vi "PH_ImageCoG_Plotter.export Data.vi"(0 "i ref in":refnum<vi>, 5 "error in (no error)":errorcluster) -> (14 "i ref out":refnum<vi>, 19 "error out":errorcluster)   [LabVIEW 2014, in "PH_ImageCoG_Plotter.lvlib"]
doc: "This VI exports data to a file"
uses:
  PH_ImageCoG_Plotter.lvlib
  PH_Basics/PH_Img_BaseClass/PH_Img_BaseClass.lvlib
  PH_Basics/PH_Common/PH_Common.lvlib
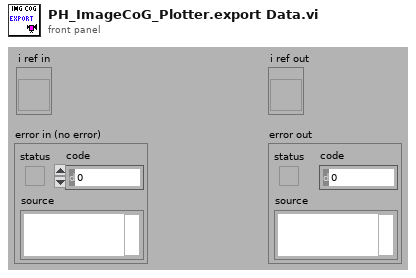
[diagram p1: front panel]
types:
  T1 = typedef "PH_ImageCoG_Plotter.lvlib/PH_ImageCoG_Plotter.i attribute.ctl" = cluster{"GUI Refs":cluster{"Delete":refnum<vi>, "Calibration status":refnum<vi>, "BI subtracted":refnum<vi>, "calc Beam Anal":refnum<vi>, "CoG - x":refnum<vi>, "CoG - y":refnum<vi>, "Type":refnum<vi>, "Center":refnum<vi>, "exp - X":refnum<vi>, "exp - Y":refnum<vi>, "Delta - X":refnum<vi>, "Delta - Y":refnum<vi>, "Available Cams":refnum<vi>, "CoG X":refnum<vi>, "CoG Y":refnum<vi>, "Delta X":refnum<vi>, "Delta Y":refnum<vi>, "Export Data":refnum<vi>, "Calibration data":refnum<vi>}, "Calibration":cluster{"Status":T2, "Calibration data":T3, "Calibration Data File":path}, "Beam Analysis":cluster{"on":bool, "exp - X":i32, "exp - Y":i32, "Type":bool, "Data":cluster{"current time":timestamp, "CoG-x":dbl, "CoG-y":dbl, "Delta-x":dbl, "Delta-y":dbl}[], "Datasets strored":i32, "Dataarray Size":i32}, "Cam instances":string[], "DIM Service Events":T4[], "Images":cluster{"Background":T7, "OP":T7, "GUI":T7}}
  T2 = typedef "PH_StatusHandler.lvlib/PH_StatusHandler.Status.ctl" = i16
  T3 = typedef "PH_ImageCalibrator.lvlib/PH_ImageCalibrator.Calibration Data.ctl" = cluster{"Date":string, "Time":string, "Cam Settings":cluster{"Cam ID":string, "Gain":dbl, "Brightness":dbl, "Shutter":dbl, "Cam Error":bool, "Mode":i32}, "Background Image":cluster{"Image":dbl[][], "Image Error":bool}, "Linear Calibration":cluster{"Calibration Factor":dbl, "not mm or mrad":bool}, "Energy Calibration":cluster{"Calibration Factor":dbl, "no mJ":bool}}
  T4 = typedef "BaseProcess.lvlib/BaseProcess.event definition.ctl" = cluster{"CAEEvtDef":T5, "Data Descriptor":T6}
  T5 = typedef "CAEObj.lvlib/CAEObj.event definition.ctl" = cluster{"URL":string, "enable":bool, "ignoreResID":bool}
  T6 = typedef "BaseProcess.lvlib/BaseProcess.descriptor string definition.ctl" = string
  T7 = typedef "IMAQ Image.ctl" = refnum<image>
  T8 = cluster{"current time":timestamp, "CoG-x":dbl, "CoG-y":dbl, "Delta-x":dbl, "Delta-y":dbl}[]
  T9 = cluster{"current time":timestamp, "CoG-x":dbl, "CoG-y":dbl, "Delta-x":dbl, "Delta-y":dbl}
  T10 = typedef "PH_Img_BaseClass.lvlib/PH_Img_BaseClass.i attribute.ctl" = cluster{"GUI Refs":T11, "Timeout Image [ms]":i32, "Default Periodic Period [ms]":i32, "Camera":cluster{"Instancename":string, "Notifier":refnum<notifier>}, "Palette":T12, "Cam Settings":cluster{"Cam ID":string, "Gain":dbl, "Brightness":dbl, "Shutter":dbl, "Cam Info Failure":bool, "Mode":i32}}
  T11 = typedef "PH_Img_BaseClass.lvlib/PH_Img_BaseClass.GUI Refs.ctl" = cluster{"Timeout":refnum<vi>, "Image":refnum<vi>, "Palette":refnum<vi>, "Timeout Set":refnum<vi>}
  T12 = typedef "PH_Img_BaseClass.lvlib/PH_Img_BaseClass.Palette.ctl" = i32
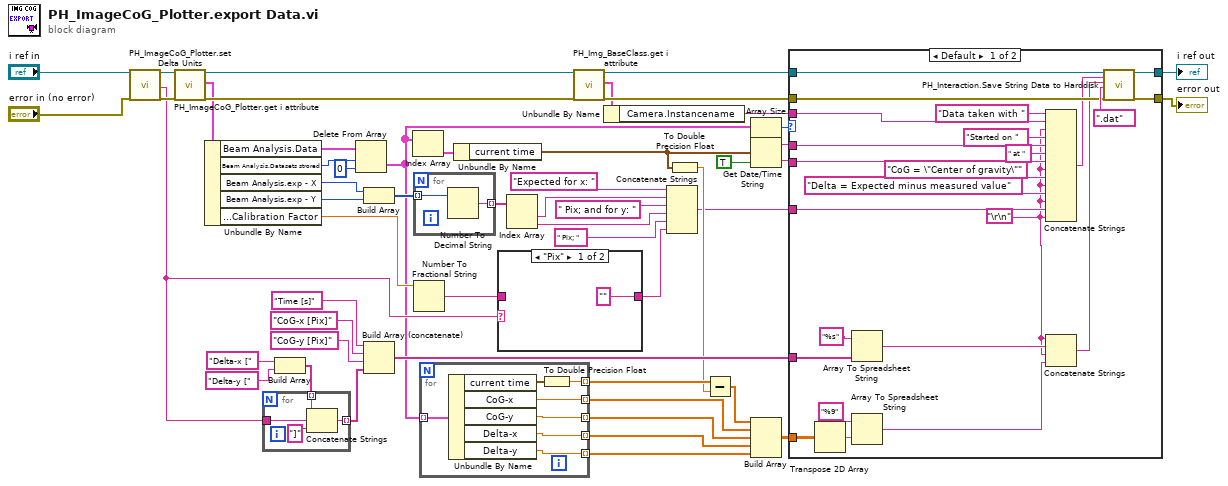
[diagram p0: block diagram]
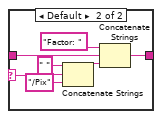
[diagram p2: hidden frame]
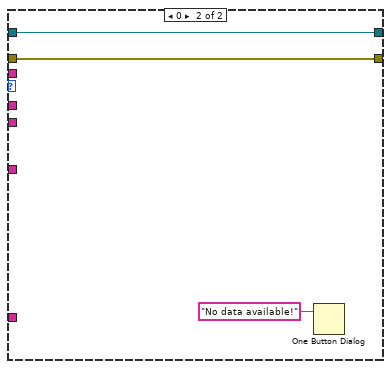
[diagram p3: hidden frame]
diagram:
  n1 = call "PH_ImageCoG_Plotter.set Delta Units.vi"("i ref in"="i ref in", "error in (no error)"="error in (no error)") -> ("i ref out"=w44:refnum<vi>, "Unit"=w10:string, "error out"=w42:errorcluster)  [unwired: 15 in]
  n2 = call "PH_ImageCoG_Plotter.get i attribute.vi"("i ref in"=w44, "error in (no error)"=w42) -> ("i ref out"=w5:refnum<vi>, "i attribute"=w51:T1, "error out"=w52:errorcluster)  [unwired: 15 in]
  n3 = Unbundle By Name(w51) -> ("Beam Analysis.Data"=w33:T8, "Beam Analysis.Datasets strored"=w8:i32, "Beam Analysis.exp - X"=w22:i32, "Beam Analysis.exp - Y"=w23:i32, "Calibration.Calibration data.Linear Calibration.Calibration Factor"=w20:dbl)
  n4 = Build Array("Delta-x [" ("element"), "Delta-y [" ("element")) -> (w35:string[])
  n5 = for {
    tunnel: w10 -> [w57]
    tunnel: w35 -> [w55] mode=indexing
    tunnel: [w54] -> w34 mode=indexing
    n6 = Concatenate Strings(w55, w57, "]" ("string")) -> (w54:string)
  }
  n7 = Delete From Array(array=w33, length=w8, index=0) -> (deleted portion=w9:T8)  [unwired: 1 out]
  n8 = Build Array(w22, w23) -> (w21:i32[])
  n9 = Build Array (concatenate)("Time [s]" ("format string"), "CoG-x [Pix]" ("element"), "CoG-y [Pix]" ("element"), w34) -> (w41:string[])
  n10 = Index Array(array=w9) -> (element=w50:T9)  [unwired: 1 in]
  n11 = for {
    tunnel: w21 -> [w59] mode=indexing
    tunnel: [w58] -> w18 mode=indexing
    n12 = Number To Decimal String(number=w59) -> (decimal integer string=w58:string)  [unwired: 1 in]
  }
  n13 = Number To Fractional String(number=w20) -> (F-format string=w12:string)  [unwired: 3 in]
  n14 = for {
    tunnel: w9 -> [w66] mode=indexing
    tunnel: [w64] -> w32 mode=indexing
    tunnel: [w63] -> w28 mode=indexing
    tunnel: [w62] -> w27 mode=indexing
    tunnel: [w61] -> w26 mode=indexing
    tunnel: [w60] -> w25 mode=indexing
    n15 = Unbundle By Name(w66) -> ("current time"=w65:timestamp, "CoG-x"=w63:dbl, "CoG-y"=w62:dbl, "Delta-x"=w61:dbl, "Delta-y"=w60:dbl)
    n16 = To Double Precision Float(number=w65) -> (double precision float=w64:dbl)
  }
  n17 = Unbundle By Name(w50) -> ("current time"=w31:timestamp)
  n18 = case shown="\"Pix\"" w10 {
    selector: w10 -> [_ w69]
    tunnel: ["" w74] -> w13
    tunnel: w12 -> [_ w72]
    frame "Pix" {
    }
    frame Default {
      n19 = Concatenate Strings(" " ("string"), w69, "/Pix" ("string")) -> (w71:string)
      n20 = Concatenate Strings("Factor: " ("string"), w72, w71) -> (w74:string)
    }
  }
  n21 = Index Array(array=w18) -> (element #1=w17:string, element #2=w15:string)  [unwired: 2 in]
  n22 = call "PH_Img_BaseClass.get i attribute.vi"("i ref in"=w5, "error in (no error)"=w52) -> ("i ref out"=w2:refnum<vi>, "i attribute"=w4:T10, "error out"=w6:errorcluster)  [unwired: 15 in]
  n23 = Unbundle By Name(w4) -> ("Camera.Instancename"=w3:string)
  n24 = Concatenate Strings("Expected for x: " ("string"), w17, " Pix; and for y: " ("string"), w15, " Pix; " ("string"), w13) -> (w11:string)
  n25 = To Double Precision Float(number=w31) -> (double precision float=w30:dbl)
  n26 = Subtract(x=w32, y=w30) -> (x-y=w29:dbl[])
  n27 = Array Size(array=w9) -> (size(s)=w46:i32)
  n28 = Get Date/Time String(seconds (now)=w31, want seconds? (F)=TRUE) -> (date string=w49:string, time string=w48:string)  [unwired: 1 in]
  n29 = Build Array(w29, w28, w27, w26, w25) -> (w24:dbl[][])
  n30 = case shown="Default" w46 {
    tunnel: w3 -> [w94 _]
    tunnel: w49 -> [w93 _]
    tunnel: w48 -> [w91 _]
    tunnel: w41 -> [w89 _]
    tunnel: w24 -> [w88 _]
    tunnel: w6 -> [w81 w100]
    tunnel: [w80 w100] -> w53
    tunnel: w11 -> [w85 _]
    tunnel: w2 -> [w83 w99]
    tunnel: [w82 w99] -> w1
    frame Default {
      w77 = "\r\n"
      n31 = Transpose 2D Array(2D array=w88) -> (transposed array=w90:dbl[][])
      n32 = Array To Spreadsheet String(array=w89, 3:"%s" ("format string")) -> (spreadsheet string=w78:string)  [unwired: 1 in]
      n33 = Array To Spreadsheet String(array=w90, 3:"%9" ("format string")) -> (spreadsheet string=w79:string)  [unwired: 1 in]
      n34 = Concatenate Strings("Data taken with " ("string"), w94, w77, "Started on ", w93, " at " ("string"), w91, w77, "CoG = \"Center of gravity\"" ("string"), w77, "Delta = Expected minus measured value" ("string"), w77, w85, w77) -> (w76:string)
      n35 = Concatenate Strings(w77, w78, w77, w79) -> (w75:string)
      n36 = call "PH_Interaction.Save String Data to Harddisk.vi"("i ref in"=w83, "Explanation (for Example: Column 1: xxx, ...)"=w76, "Data (for example: Columns)"=w75, "file name extension"=".dat" ("file name extinction"), "error in (no error)"=w81) -> ("i ref out"=w82:refnum<vi>, "error out"=w80:errorcluster)  [unwired: 12 in, 1 out]
    }
    frame 0 {
      n37 = One Button Dialog(message="No data available!") -> ()  [unwired: 1 in, 1 out]
    }
  }
  "error out" <- w53
  "i ref out" <- w1
